vi "Parse.vi"(8 "Error In":errorcluster, 11 "object in":refnum<class "2021_21.lvclass">) -> (0 "Error Out":errorcluster, 3 "object out":refnum<class "2021_21.lvclass">)   [LabVIEW 2020, in "2021_21.lvclass"]
uses:
  2021_21.lvclass
  2021_21.lvclass/2021_21.ctl
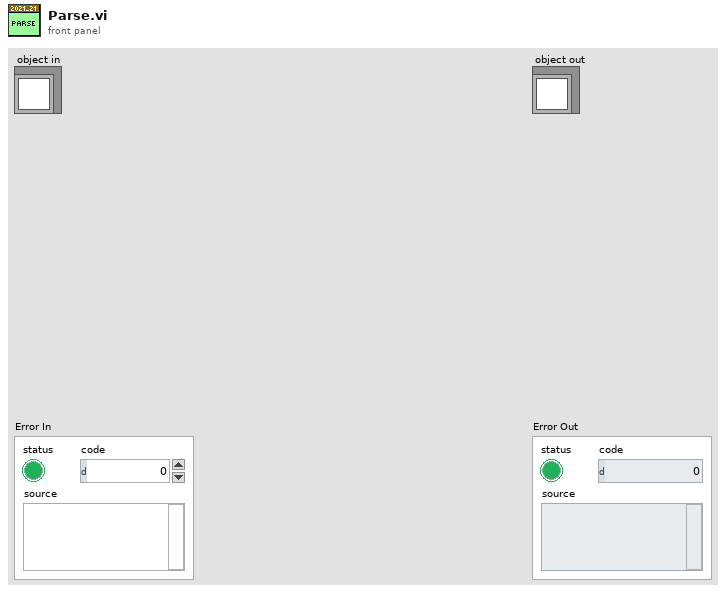
[diagram p1: front panel]
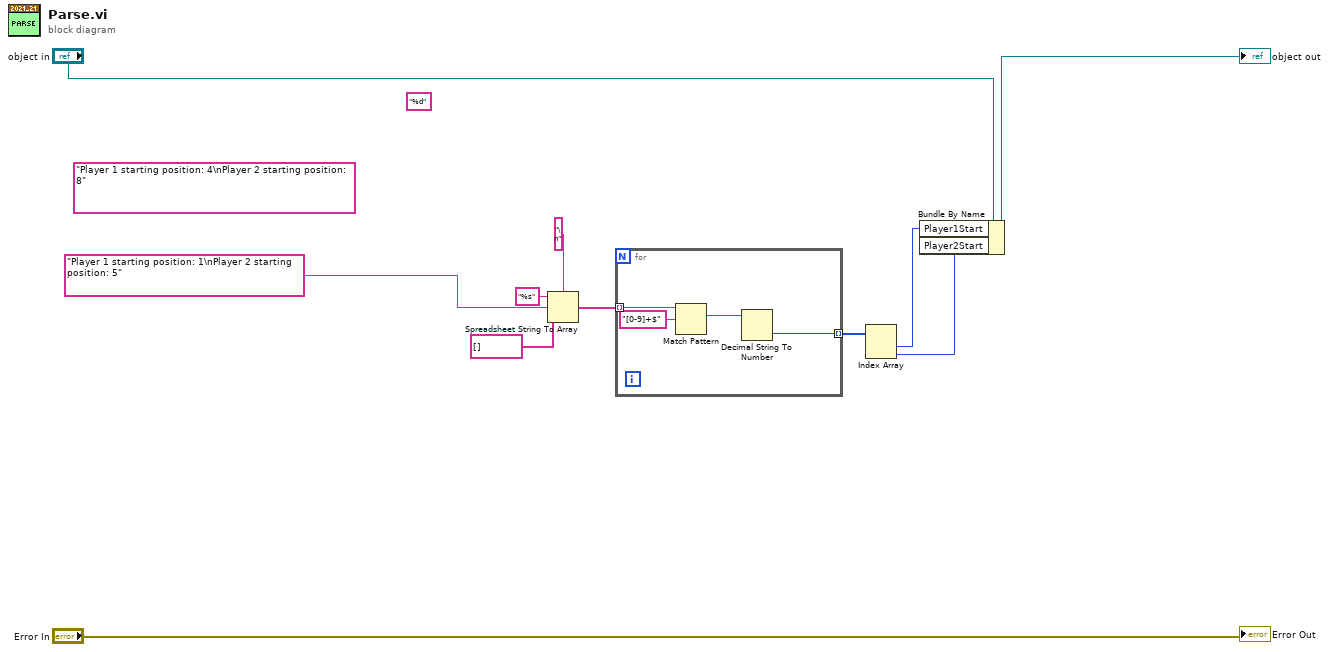
[diagram p0: block diagram]
diagram:
  (unwired) "Player 1 starting position: 4\nPlayer 2 starting position: 8" ("PuzzleInput")
  (unwired) "%d" ("format string")
  n1 = Spreadsheet String To Array(delimiter (Tab)="\n", format string="%s", spreadsheet string="Player 1 starting position: 1\nPlayer 2 starting position: 5" ("PuzzleInput"), array type (2D Dbl)=string[] []) -> (array=w5:string[])
  n2 = for {
    tunnel: w5 -> [w15] mode=indexing
    tunnel: [w12] -> w4 mode=indexing
    n3 = Match Pattern(string=w15, regular expression="[0-9]+$") -> (match substring=w13:string)  [unwired: 1 in, 3 out]
    n4 = Decimal String To Number(string=w13) -> (number=w12:i32)  [unwired: 2 in, 1 out]
  }
  n5 = Index Array(array=w4) -> (element #1=w3:i32, element #2=w2:i32)  [unwired: 2 in]
  n6 = Bundle By Name(cluster="object in", "Player1Start"=w3, "Player2Start"=w2) -> (→"object out":refnum<class "2021_21.lvclass">)
  "Error Out" <- "Error In"
